vi "Bin counts together.vi"(8 "bin width (unitless, assumed nm)":dbl, 9 "center wavelength \nof last bin  (unitless, assumed nm)":dbl, 10 "center wavelength \nof first bin (unitless, assumed nm)":dbl, 11 "Array of wavelengths \nand counts (unitless, assumed nm)":dbl[][](array[numeric])) -> (0 "array of number of pixels\nused for the total bin counts":i32[](array[numeric]), 3 "binned array of wavelengths \nand counts (unitless, assumed nm)":dbl[][](array[numeric]))   [LabVIEW 2017]
panel:
  out "temp array of \ncounts for this bin":dbl[](array[numeric])
  out "center wavelength\nof ith bin":dbl
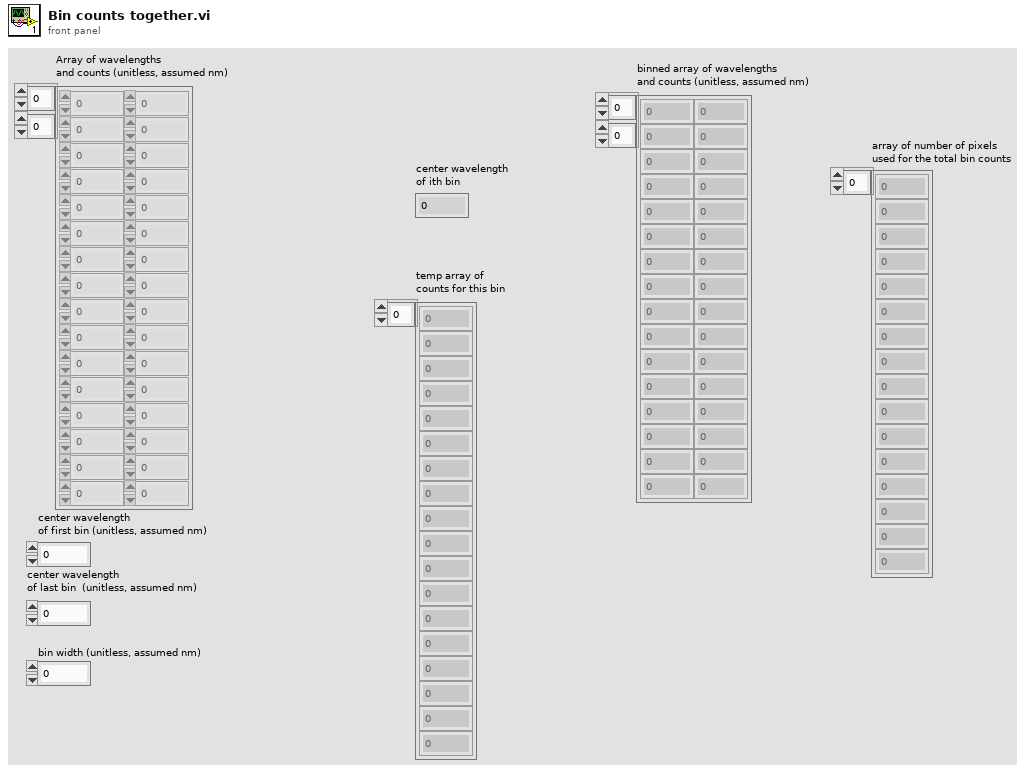
[diagram p1: front panel]
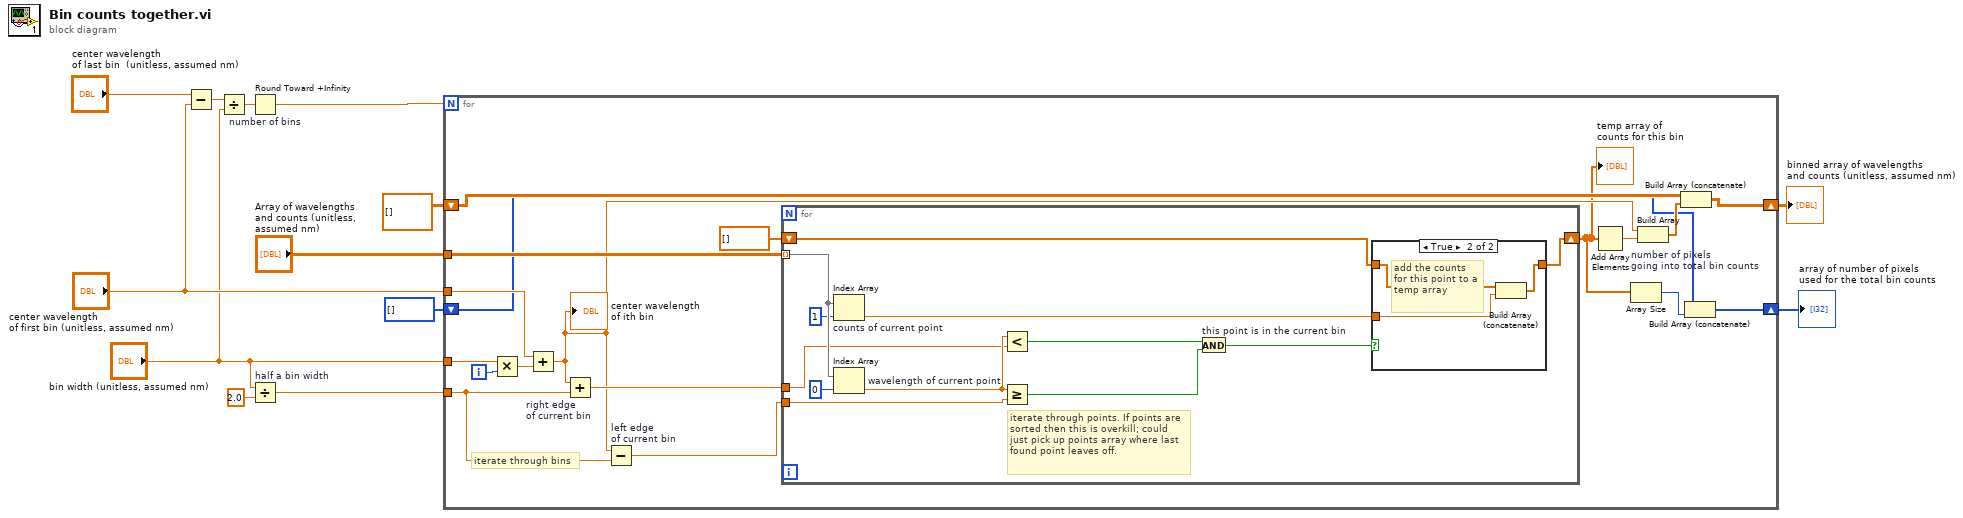
[diagram p0: block diagram]
diagram:
  n1 = Subtract(x="center wavelength \nof last bin  (unitless, assumed nm)", y="center wavelength \nof first bin (unitless, assumed nm)") -> (x-y=w13:dbl)
  n2 = Divide(x=w13, y="bin width (unitless, assumed nm)") -> (x/y=w12:dbl)
  n3 = Round Toward +Infinity "number of bins"(x=w12) -> (ceil(x): smallest int >= x=w11:dbl)
  n4 = Divide "half a bin width"(x="bin width (unitless, assumed nm)", y=2.0) -> (x/y=w9:dbl)
  n5 = for {
    N: w11 -> [_]
    tunnel: "center wavelength \nof first bin (unitless, assumed nm)" -> [w28]
    tunnel: "bin width (unitless, assumed nm)" -> [w30]
    tunnel: w9 -> [w27]
    tunnel: "Array of wavelengths \nand counts (unitless, assumed nm)" -> [w26]
    shift-right: [w18] -> w7
    shift-left: dbl[][] [] ("binned array of wavelengths/counts (unitless, assumed nm) 2") -> [w20]
    shift-right: [w15] -> w1
    shift-left: i32[] [] -> [w14]
    i -> [w31]
    # "iterate through bins"
    n6 = Multiply(x=w30, y=w31) -> (x*y=w29:dbl)
    n7 = Add(x=w28, y=w29) -> (x+y=w22:dbl)
    "center wavelength\nof ith bin" <- w22
    n8 = Add "right edge \nof current bin"(x=w22, y=w27) -> (x+y=w25:dbl)
    n9 = Subtract "left edge \nof current bin"(x=w22, y=w27) -> (x-y=w24:dbl)
    n10 = for {
      tunnel: w26 -> [w42] mode=indexing
      tunnel: w25 -> [w39]
      tunnel: w24 -> [w38]
      shift-right: [w32] -> w17
      shift-left: dbl[] [] ("temp array of counts for this bin") -> [w34]
      # "iterate through points. If points are sorted then this is overkill; could just pick up points array where last found point leaves off."
      n11 = Index Array "counts of current point"(array=w42, index=1) -> (element=w33:dbl)
      n12 = Index Array "wavelength of current point"(array=w42, index=0) -> (element=w40:dbl)
      n13 = Less?(x=w40, y=w39) -> (x < y?=w37:bool)
      n14 = Greater Or Equal?(x=w40, y=w38) -> (x >= y?=w36:bool)
      n15 = And "this point is in the current bin"(x=w37, y=w36) -> (x .and. y?=w35:bool)
      n16 = case shown="True" w35 {
        tunnel: w34 -> [w44 w47]
        tunnel: w33 -> [_ w46]
        tunnel: [w44 w45] -> w32
        frame False {
        }
        frame True {
          # "add the counts for this point to a temp array"
          n17 = Build Array (concatenate)(w47, w46) -> (w45:dbl[])
        }
      }
    }
    "temp array of \ncounts for this bin" <- w17
    n18 = Add Array Elements(numeric array=w17) -> (sum=w21:dbl)
    n19 = Array Size "number of pixels \ngoing into total bin counts"(array=w17) -> (size(s)=w16:i32)
    n20 = Build Array(w22, w21) -> (w19:dbl[])
    n21 = Build Array (concatenate)(w20, w19) -> (w18:dbl[][])
    n22 = Build Array (concatenate)(w14, w16) -> (w15:i32[])
  }
  "binned array of wavelengths \nand counts (unitless, assumed nm)" <- w7
  "array of number of pixels\nused for the total bin counts" <- w1
